vi "Set_Pressure.vi"(9 "Current Out Mode":bool=TRUE, 10 "Set Pressure (PSI)":dbl) -> (2 "Current Sent (mA)":dbl)   [LabVIEW 2019]
panel:
  # "The Equilibar differential pressure sensor takes \nan analog current input of 4-20mA and scales \npressure against full scale (1000psi) for this case"
  # "If set to false, \nSets Output current to 0A"
  # "0 Current"
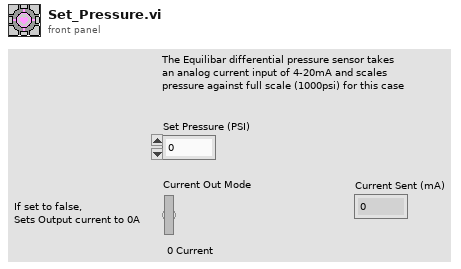
[diagram p1: front panel]
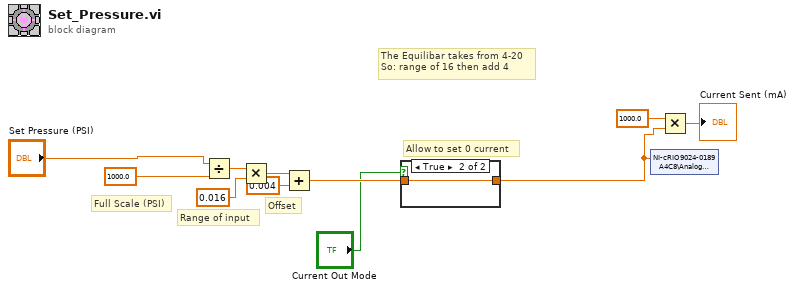
[diagram p0: block diagram]
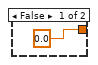
[diagram p2: hidden frame]
diagram:
  # "Allow to set 0 current"
  # "Offset"
  # "Range of input"
  # "The Equilibar takes from 4-20\nSo: range of 16 then add 4"
  # "Full Scale (PSI)"
  n1 = Divide(x="Set Pressure (PSI)", y=1000.0) -> (x/y=w10:dbl)
  n2 = Multiply(x=w10, y=0.016) -> (x*y=w8:dbl)
  n3 = Add(x=w8, y=0.004) -> (x+y=w6:dbl)
  n4 = case shown="True" "Current Out Mode" {
    tunnel: w6 -> [_ w13]
    tunnel: [0.0 w13] -> w3
    frame False {
    }
    frame True {
    }
  }
  n5 = shared-variable "NI-cRIO9024-0189A4C8\\Analog Current Out\\AO0"(w3) -> ()  [unwired: 1 in, 1 out]
  n6 = Multiply(x=1000.0, y=w3) -> (x*y=→"Current Sent (mA)":dbl)
